vi "Hex_String_to_Binary_String.vi"(4 "bitness":enum16{"8", "16", "32", "64"}(ring), 5 "Hexadecimal String":string="FF") -> (0 "number":u64, 1 "Hex String":string, 2 "Binary String":string)   [LabVIEW 2025]
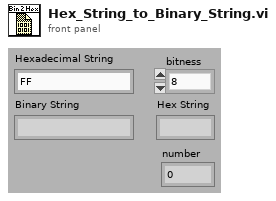
[diagram p1: front panel]
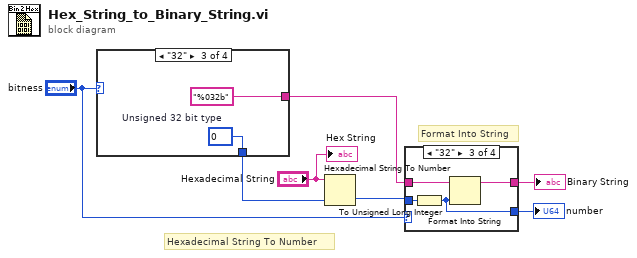
[diagram p0: block diagram]
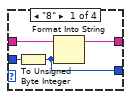
[diagram p2: hidden frame]
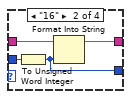
[diagram p3: hidden frame]
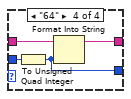
[diagram p4: hidden frame]
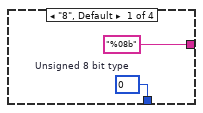
[diagram p5: hidden frame]
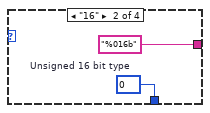
[diagram p6: hidden frame]
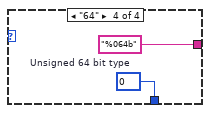
[diagram p7: hidden frame]
diagram:
  # "Format Into String"
  # "Hexadecimal String To Number"
  n1 = case shown="\"32\"" "bitness" {
    tunnel: ["%08b" ("format string") "%016b" ("format string") "%032b" ("format string") "%064b" ("format string")] -> w4
    tunnel: [w8 w10 w12 w14] -> w3
    frame "8", Default {
      w8 = u8 0  # Unsigned 8 bit type
    }
    frame "16" {
      w10 = u16 0  # Unsigned 16 bit type
    }
    frame "32" {
      w12 = u32 0  # Unsigned 32 bit type
    }
    frame "64" {
      w14 = u64 0  # Unsigned 64 bit type
    }
  }
  n2 = Hexadecimal String To Number(string="Hexadecimal String", default (0uL)=w3) -> (number=w7:u64)  [unwired: 1 in, 1 out]
  n3 = case shown="\"32\"" "bitness" {
    tunnel: w7 -> [w19 w23 w27 w31]
    tunnel: [w18 w22 w26 w30] -> w6
    tunnel: w4 -> [w17 w21 w25 w29]
    tunnel: [w16 w20 w24 w28] -> w1
    frame "8" {
      n4 = To Unsigned Byte Integer(number=w19) -> (unsigned 8bit integer=w16:u8)
      n5 = Format Into String(format string=w17, w16) -> (resulting string=w18:string)  [unwired: 2 in, 1 out]
    }
    frame "16" {
      n6 = To Unsigned Word Integer(number=w23) -> (unsigned 16bit integer=w20:u16)
      n7 = Format Into String(format string=w21, w20) -> (resulting string=w22:string)  [unwired: 2 in, 1 out]
    }
    frame "32" {
      n8 = To Unsigned Long Integer(number=w27) -> (unsigned 32bit integer=w24:u32)
      n9 = Format Into String(format string=w25, w24) -> (resulting string=w26:string)  [unwired: 2 in, 1 out]
    }
    frame "64" {
      n10 = To Unsigned Quad Integer(1:w31) -> (0:w28:u64)
      n11 = Format Into String(format string=w29, w28) -> (resulting string=w30:string)  [unwired: 2 in, 1 out]
    }
  }
  "Binary String" <- w6
  "number" <- w1
  "Hex String" <- "Hexadecimal String"
